vi "Global Queue Ref.vi"(7 "Module":T2, 8 "error in (no error)":errorcluster, 11 "Module Name":string) -> (0 "error out":errorcluster, 3 "queue out":T1)   [LabVIEW 2019, in "Message Queue.lvlib"]
uses:
  Message Queue.lvlib
  Module Name.ctl
  Shared/TypeDefs/Message Queue Ref.ctl
  Shared/TypeDefs/Message Queue Type.ctl
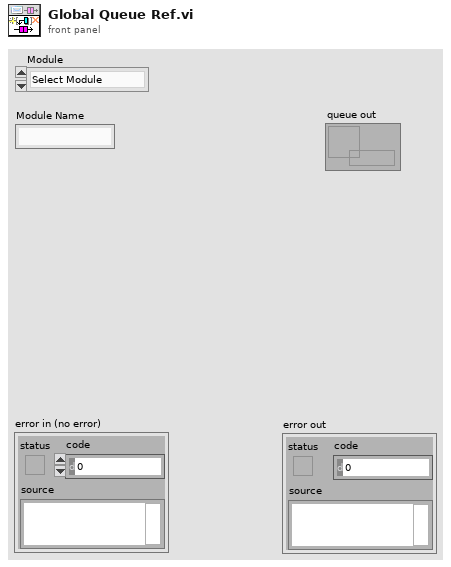
[diagram p1: front panel]
types:
  T1 = typedef "Message Queue Ref.ctl" = refnum<queue>
  T2 = typedef "Message Queue.lvlib/Module Name.ctl" = enum16{"Select Module", "Main", "Status"}
  T3 = typedef "Message Queue Type.ctl" = cluster{"Custom State Name":string, "Defined State Name":variant, "Call Chain":string[], "Message Data":variant}
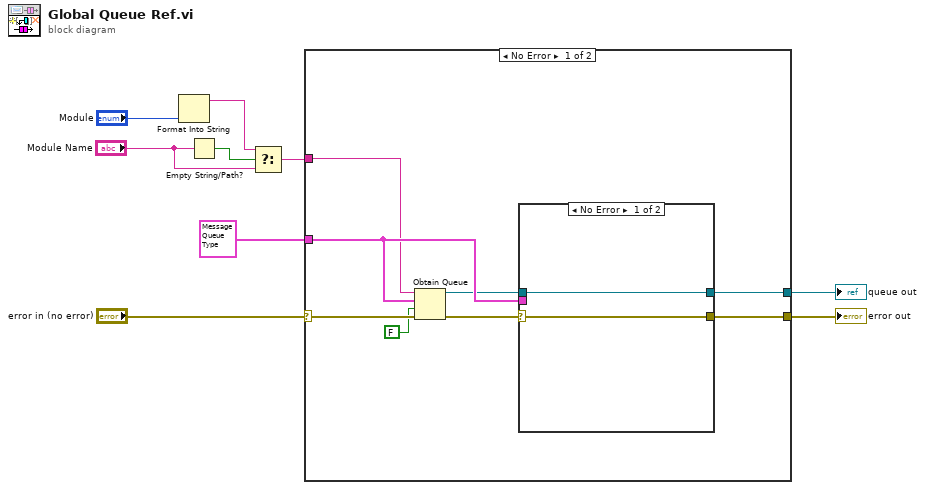
[diagram p0: block diagram]
diagram:
  n1 = Format Into String("Module") -> (resulting string=w5:string)  [unwired: 3 in, 1 out]
  n2 = Empty String/Path?(string/path="Module Name") -> (empty?=w6:bool)
  n3 = Select(t=w5, s=w6, f="Module Name") -> (s? t:f=w4:string)
  n4 = case shown="No Error" "error in (no error)" {
    selector: "error in (no error)" -> [w14 w21]
    tunnel: T3 {"Custom State Name"="", "Defined State Name"=variant(i32 0), "Call Chain"=[], "Message Data"=variant} ("Message Data") -> [w17 _]
    tunnel: [w16 w21] -> w9
    tunnel: w4 -> [w15 _]
    tunnel: [w10 _] -> w1
    frame No Error {
      n5 = Obtain Queue(name (unnamed)=w15, element data type=w17, create if not found? (T)=FALSE, error in (no error)=w14) -> (queue out=w13:refnum<queue>, error out=w11:errorcluster)  [unwired: 1 in, 1 out]
      n6 = case shown="No Error" w11 {
        selector: w11 -> [w18 w20]
        tunnel: [w18 w20] -> w16
        tunnel: w13 -> [w19 _]
        tunnel: w17 -> [_ _]
        tunnel: [w19 _] -> w10
        frame No Error {
        }
        frame Error {
        }
      }
    }
    frame Error {
    }
  }
  "error out" <- w9
  "queue out" <- w1
